vi "CAPTH-Config Channels.vi"(0 "EAR":i32(ring) items=["RIGHT", "LEFT", "ALTERNATE"], 11 "error in (no error)":errorcluster) -> (3 "active ears":i32[](array[numeric]), 4 "AO channels":u16[](array[numeric]), 6 "AI channels":u16[](array[numeric]), 15 "error out":errorcluster)   [LabVIEW 2020]
uses:
  epl-vi-lib/Connection VIs/Type Defs/Output sources.ctl
  epl-vi-lib/Connection VIs/Type Defs/Input sources.ctl
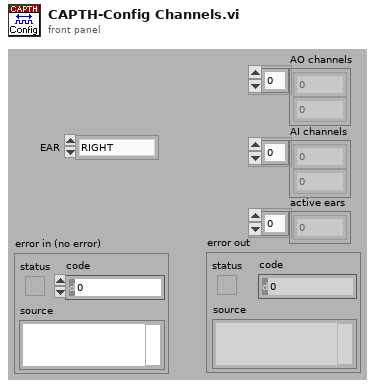
[diagram p1: front panel]
types:
  T1 = typedef "Input sources.ctl" = u16
  T2 = typedef "Output sources.ctl" = u16
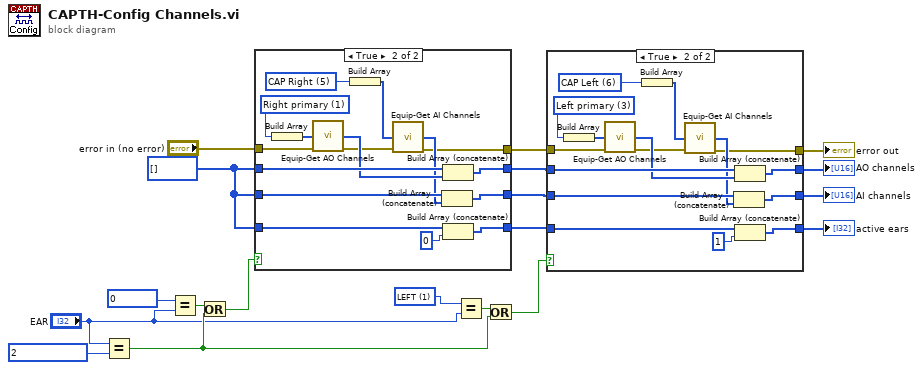
[diagram p0: block diagram]
diagram:
  w9 = 1 items=["RIGHT", "LEFT", "ALTERNATE"] ("EAR")
  w18 = u16[] [] ("appended array")
  n1 = Equal?(x="EAR", y=2 ("EAR")) -> (x = y?=w11:bool)
  n2 = Equal?(x=0 ("EAR"), y="EAR") -> (x = y?=w17:bool)
  n3 = Or(x=w17, y=w11) -> (x .or. y?=w16:bool)
  n4 = case shown="True" w16 {
    tunnel: w18 -> [w23 w39]
    tunnel: [w23 w38] -> w7
    tunnel: w18 -> [w22 w37]
    tunnel: [w22 w36] -> w6
    tunnel: w18 -> [w21 w35]
    tunnel: [w21 w34] -> w5
    tunnel: "error in (no error)" -> [w20 w31]
    tunnel: [w20 w24] -> w13
    frame False {
    }
    frame True {
      w27 = T1 5 items=["--unused--", "Probe Mic Right", "Probe Mic Left", "Cal Mic", "ABR", "CAP Right", "CAP Left", "Startle piezo", "Temperature", "Heart rate"] ("Ring")
      w33 = T2 1 items=["--unused--", "Right primary", "Right secondary", "Left primary", "Left secondary", "Shocks", "Startle", "Background"] ("Ring")
      n5 = Build Array(w33) -> (w32:T2[])
      n6 = call "Equip-Get AO Channels.vi"("Outputs"=w32, "error in (no error)"=w31) -> ("AO Channels"=w30:i32[], "error out"=w29:errorcluster)  [unwired: 12 in]
      n7 = Build Array(w27) -> (w26:T1[])
      n8 = call "Equip-Get AI Channels.vi"("Inputs"=w26, "error in (no error)"=w29) -> ("AI Channels"=w25:i32[], "error out"=w24:errorcluster)  [unwired: 12 in]
      n9 = Build Array (concatenate)(w37, w25) -> (w36:i32[])
      n10 = Build Array (concatenate)(w39, w30) -> (w38:i32[])
      n11 = Build Array (concatenate)(w35, 0) -> (w34:i32[])
    }
  }
  n12 = Equal?(x=w9, y="EAR") -> (x = y?=w12:bool)
  n13 = Or(x=w12, y=w11) -> (x .or. y?=w8:bool)
  n14 = case shown="True" w8 {
    tunnel: w7 -> [w43 w59]
    tunnel: [w43 w58] -> w2
    tunnel: w6 -> [w42 w57]
    tunnel: [w42 w56] -> w3
    tunnel: w5 -> [w41 w55]
    tunnel: [w41 w54] -> w4
    tunnel: w13 -> [w40 w51]
    tunnel: [w40 w44] -> w1
    frame False {
    }
    frame True {
      w47 = T1 6 items=["--unused--", "Probe Mic Right", "Probe Mic Left", "Cal Mic", "ABR", "CAP Right", "CAP Left", "Startle piezo", "Temperature", "Heart rate"] ("Ring")
      w53 = T2 3 items=["--unused--", "Right primary", "Right secondary", "Left primary", "Left secondary", "Shocks", "Startle", "Background"] ("Ring")
      n15 = Build Array(w53) -> (w52:T2[])
      n16 = call "Equip-Get AO Channels.vi"("Outputs"=w52, "error in (no error)"=w51) -> ("AO Channels"=w50:i32[], "error out"=w49:errorcluster)  [unwired: 12 in]
      n17 = Build Array(w47) -> (w46:T1[])
      n18 = call "Equip-Get AI Channels.vi"("Inputs"=w46, "error in (no error)"=w49) -> ("AI Channels"=w45:i32[], "error out"=w44:errorcluster)  [unwired: 12 in]
      n19 = Build Array (concatenate)(w57, w45) -> (w56:i32[])
      n20 = Build Array (concatenate)(w59, w50) -> (w58:i32[])
      n21 = Build Array (concatenate)(w55, 1) -> (w54:i32[])
    }
  }
  "error out" <- w1
  "AO channels" <- w2
  "AI channels" <- w3
  "active ears" <- w4
